vi "gmxl_PolyParse.vi"   [LabVIEW 2011, in "Third Party VIs.lvlib" / "GXML.lvlib"]
doc: "Using a custom XML schema, this VI converts an XML string into a user specified LabVIEW data type. The data structure is defined by the input <b>TypeDesc</b> and its elements must have the same name and hierarchy as the elements in the XML string."
uses:
  GXML.lvlib
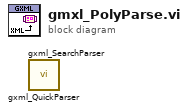
[diagram p0: block diagram]
diagram:
  n1 = call "gxml_QuickParser.vi"() -> ()  [unwired: 10 in, 2 out]
  n2 = call "gxml_SearchParser.vi"() -> ()  [unwired: 10 in, 2 out]
